vi "Obtain Queue.vi"(7 "Q Name":string, 8 "error in":errorcluster, 10 "Q Element data type":refnum<class "IMessagePayload.lvclass">, 11 "QueueMessageTransport in":refnum<class "QueueMessageTransport.lvclass">) -> (0 "error out":errorcluster, 3 "QueueMessageTransport out":refnum<class "QueueMessageTransport.lvclass">)   [LabVIEW 2016, in "QueueMessageTransport.lvclass"]
doc: "This public method creates a Queue reference\n\n**Author: Stas Legedza"
uses:
  QueueMessageTransport.lvclass
  IMessagePayload/IMessagePayload.lvclass
  QueueMessageTransport.lvclass/QueueMessageTransport.ctl
panel:
  # "INPUTS"
  # "OUTPUTS"
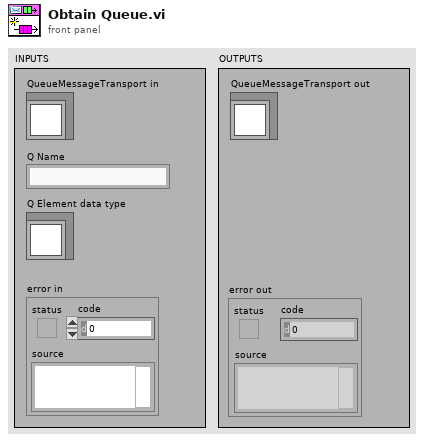
[diagram p1: front panel]
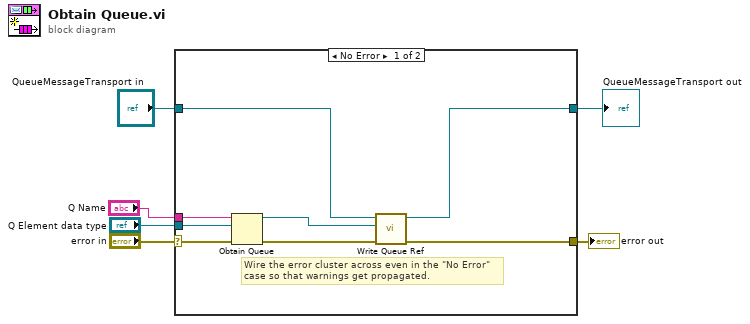
[diagram p0: block diagram]
diagram:
  n1 = case shown="No Error" "error in" {
    selector: "error in" -> [w13 w16]
    tunnel: [w12 w16] -> w5
    tunnel: [w8 w15] -> w3
    tunnel: "QueueMessageTransport in" -> [w11 w15]
    tunnel: "Q Name" -> [w14 _]
    tunnel: "Q Element data type" -> [w7 _]
    frame No Error {
      # "Wire the error cluster across even in the \"No Error\"\ncase so that warnings get propagated."
      n2 = Obtain Queue(name (unnamed)=w14, element data type=w7, error in (no error)=w13) -> (queue out=w9:refnum<queue>, error out=w10:errorcluster)  [unwired: 2 in, 1 out]
      n3 = call "Write Queue Ref.vi"("error in"=w10, "Queue Ref"=w9, "QueueMessageTransport in"=w11) -> ("error out"=w12:errorcluster, "QueueMessageTransport out"=w8:refnum<class "QueueMessageTransport.lvclass">)  [unwired: 7 in]
    }
    frame Error {
    }
  }
  "error out" <- w5
  "QueueMessageTransport out" <- w3
